vi "hold_time.vi"(1 "Sample?":bool, 2 "Hold Time in Seconds":i16) -> ()   [LabVIEW 2010]
uses:
  <vilib>/Utility/file.llb/Write To Spreadsheet File (DBL).vi
  <vilib>/Utility/file.llb/Write To Spreadsheet File (string).vi
panel:
  in  "Sample (or CRM) ID":string
  in  "File Path in":path
  in  "Record Hold File?":bool
  out "emf":ext(graph)
  in  "Stop Hold":bool=TRUE
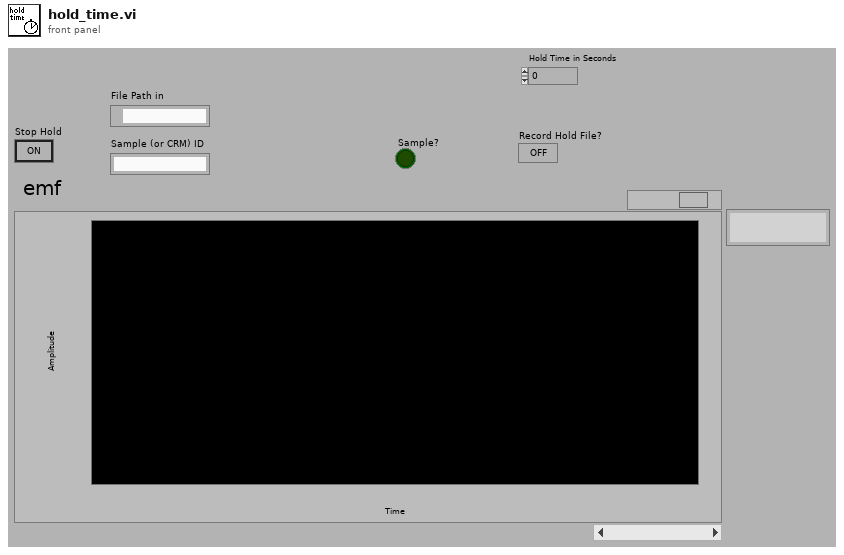
[diagram p1: front panel]
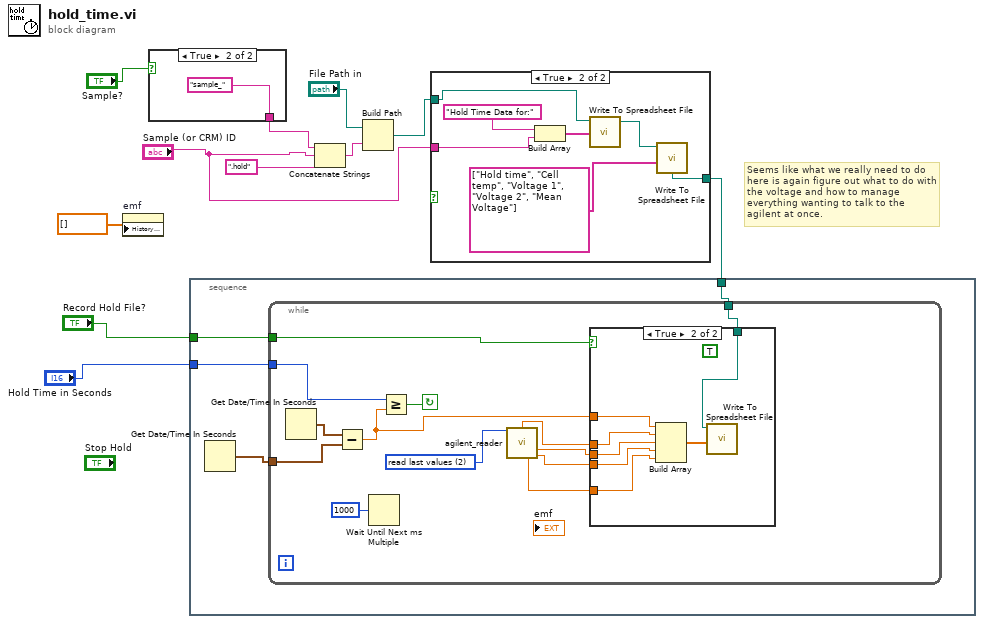
[diagram p0: block diagram]
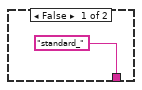
[diagram p3: hidden frame]
diagram:
  # "Seems like what we really need to do here is again figure out what to do with the voltage and how to manage everything wanting to talk to the agilent at once."
  n1 = property on="emf" class="WFChart (strict)"("History Data"=ext[] []) -> ()  [unwired: 2 in, 2 out]
  n2 = case shown="True" "Sample?" {
    tunnel: ["standard_" "sample_"] -> w5
    frame False {
    }
    frame True {
    }
  }
  n3 = Concatenate Strings(w5, "Sample (or CRM) ID", ".hold" ("string")) -> (w10:string)
  n4 = Build Path(base path="File Path in", name or relative path=w10) -> (appended path=w3:path)
  n5 = case shown="True" {
    selector: _ -> [_ _]
    tunnel: w3 -> [w14 w18]
    tunnel: [w14 w21] -> w2
    tunnel: "Sample (or CRM) ID" -> [_ w17]
    frame False {
    }
    frame True {
      n6 = Build Array("Hold Time Data for:", w17) -> (w15:string[])
      n7 = call-poly <vilib>:"Write To Spreadsheet File.vi"("1D data"=w15, "file path (dialog if empty)"=w18) -> ("new file path (Not A Path if cancelled)"=w19:path)  [unwired: 6 in]
      n8 = call-poly <vilib>:"Write To Spreadsheet File.vi"("1D data"=string[] ["Hold time", "Cell temp", "Voltage 1", "Voltage 2", "Mean Voltage"], "file path (dialog if empty)"=w19) -> ("new file path (Not A Path if cancelled)"=w21:path)  [unwired: 6 in]
    }
  }
  n9 = stacked-sequence {
    tunnel: w2 -> [w25]
    tunnel: "Hold Time in Seconds" -> [w24]
    tunnel: "Record Hold File?" -> [w22]
    frame #0 {
      n10 = Get Date/Time In Seconds() -> (seconds since 1Jan1904=w23:timestamp)
      n11 = while {
        tunnel: w24 -> [w36]
        tunnel: w23 -> [w38]
        tunnel: w25 -> [w34]
        tunnel: w22 -> [w32]
        stop <- w35 continue-if-true
        w31 = u8 2 items=["read new values"=1, "read last values "=2] ("Action")
        n12 = Get Date/Time In Seconds() -> (seconds since 1Jan1904=w33:timestamp)
        n13 = Subtract(x=w33, y=w38) -> (x-y=w29:dbl)
        n14 = Wait Until Next ms Multiple(millisecond multiple=u32 1000) -> ()  [unwired: 1 out]
        n15 = Greater Or Equal?(x=w36, y=w29) -> (x >= y?=w35:bool)
        n16 = call "agilent_reader.vi"("Action"=w31) -> ("Cell Temp"=w30:dbl, "Voltage 1"=w28:dbl, "Average Voltage"=w26:dbl, "Voltage 2"=w27:dbl)  [unwired: 5 in, 6 out]
        n17 = case shown="True" w32 {
          tunnel: w34 -> [_ w45]
          tunnel: w30 -> [_ w43]
          tunnel: w29 -> [_ w44]
          tunnel: w28 -> [_ w42]
          tunnel: w27 -> [_ w41]
          tunnel: w26 -> [_ w40]
          frame False {
          }
          frame True {
            (unwired) TRUE ("append to file? (new file:F)")
            n18 = Build Array(w44, w43, w42, w41, w40) -> (w39:dbl[])
            n19 = call-poly <vilib>:"Write To Spreadsheet File.vi"("1D data"=w39, "file path (dialog if empty)"=w45) -> ()  [unwired: 6 in, 1 out]
          }
        }
      }
    }
  }
